vi "Read Mixed Modules at Indexes.vi"(5 "Indexes":i32[](array[numeric]), 7 "R/W Case":T1, 8 "error in (no error)":errorcluster, 10 "Async in in":T13, 11 "RSI Modules in in":T2[](array[typedef]) {"Module Config Data"."Config Block Data Refs"."Data Reference" format="%.0x"; "CDOutput Data"."BD Refs"."Data Reference" format="%.0x"; "CDInput Data"."BD Refs"."Data Reference" format="%.0x"; "VS ref" format="%.0x"}) -> (0 "error out":errorcluster, 2 "Async in out":T13, 3 "RSI Modules in out":T2[](array[typedef]) {"Module Config Data"."Config Block Data Refs"."Data Reference" format="%.0x"; "CDOutput Data"."BD Refs"."Data Reference" format="%.0x"; "CDInput Data"."BD Refs"."Data Reference" format="%.0x"; "VS ref" format="%.0x"})   [LabVIEW 2016, in "Scan Engine Custom Device.lvlib"]
uses:
  Scan Engine Custom Device.lvlib
  Type Defs/Async Command.ctl
  Type Defs/Async State.ctl
  Type Defs/Async Status.ctl
  Type Defs/Async Data.ctl
  <vilib>/NI Veristand/Custom Device API/Custom Device Item Ref.ctl
  <vilib>/NI Veristand/Custom Device API/Custom Device API.lvlib
  <vilib>/NI Veristand/Custom Device API/Data Reference.ctl
  <vilib>/NI Veristand/Custom Device API/Block Data Reference.ctl
  Type Defs/Input Data.ctl
  Type Defs/Output Data.ctl
  Modules.lvlibp/RSI Module/Channel Type.ctl
  Modules.lvlibp/RSI Module/RSI Module.lvclass
  Modules.lvlibp/RSI Module/Module Models.ctl
  Type Defs/Module Config Data.ctl
  Type Defs/Mixed IO.ctl
  Type Defs/Open Module IOVs.ctl
  Type Defs/RSI Module Data.ctl
  Type Defs/RW Case.ctl
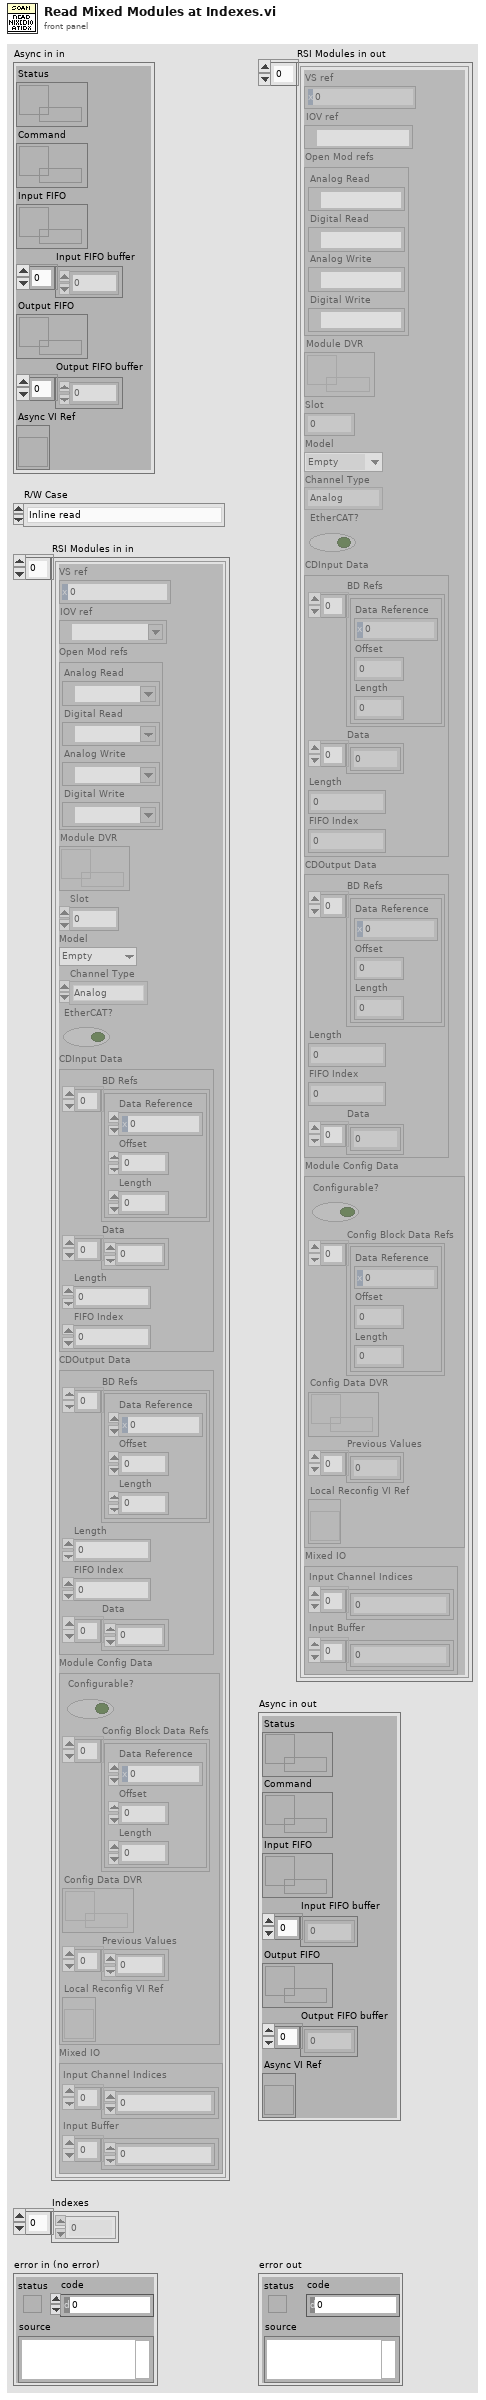
[diagram p1: front panel]
types:
  T1 = typedef "Scan Engine Custom Device.lvlib/RW Case.ctl" = enum16{"Inline read", "Inline write", "Async - Inline loop read", "Async - Inline loop write", "Async loop (read/write)"}
  T2 = typedef "Scan Engine Custom Device.lvlib/RSI Module Data.ctl" = cluster{"VS ref":T3, "IOV ref":refnum<k21>, "Open Mod refs":T4, "Module DVR":refnum<data-value>, "Slot":u32, "Model":T5, "Channel Type":T6, "EtherCAT?":bool, "CDInput Data":T7, "CDOutput Data":T10, "Module Config Data":T11, "Mixed IO":T12}
  T3 = typedef "Custom Device API.lvlib/Custom Device Item Ref.ctl" = u64
  T4 = typedef "Scan Engine Custom Device.lvlib/Open Module IOVs.ctl" = cluster{"Analog Read":refnum<k21>, "Digital Read":refnum<k21>, "Analog Write":refnum<k21>, "Digital Write":refnum<k21>}
  T5 = typedef "Modules.lvlibp/RSI Module.lvclass/Module Models.ctl" = enum16{"Empty", "NI 9201", "NI 9203", "NI 9205", "NI 9206", "NI 9207", "NI 9208", "NI 9211", "NI 9213", "NI 9214", "NI 9215", "NI 9217", "NI 9219", "NI 9221", "NI 9225", "NI 9227", "NI 9229", "NI 9233", "NI 9234", "NI 9235", "NI 9236", "NI 9237", "NI 9239", "NI 9263", "NI 9264", "NI 9265", "NI 9269", "NI 9375", "NI 9401", "NI 9402", "NI 9403", "NI 9411", "NI 9421", "NI 9422", "NI 9423", "NI 9425", "NI 9426", "NI 9435", "NI 9472", "NI 9474", "NI 9475", "NI 9476", "NI 9477", "NI 9478", "NI 9481", "NI 9482", "NI 9485"}
  T6 = typedef "Modules.lvlibp/RSI Module.lvclass/Channel Type.ctl" = enum16{"Analog", "Digital"}
  T7 = typedef "Scan Engine Custom Device.lvlib/Input Data.ctl" = cluster{"BD Refs":T8[], "Data":dbl[], "Length":i32, "FIFO Index":i32}
  T8 = typedef "Custom Device API.lvlib/Block Data Reference.ctl" = cluster{"Data Reference":T9, "Offset":u64, "Length":u64}
  T9 = typedef "Custom Device API.lvlib/Data Reference.ctl" = i32
  T10 = typedef "Scan Engine Custom Device.lvlib/Output Data.ctl" = cluster{"BD Refs":T8[], "Length":i32, "FIFO Index":i32, "Data":dbl[]}
  T11 = typedef "Scan Engine Custom Device.lvlib/Module Config Data.ctl" = cluster{"Configurable?":bool, "Config Block Data Refs":T8[], "Config Data DVR":refnum<data-value>, "Previous Values":dbl[], "Local Reconfig VI Ref":refnum<vi>}
  T12 = typedef "Scan Engine Custom Device.lvlib/Mixed IO.ctl" = cluster{"Input Channel Indices":i32[], "Input Buffer":dbl[]}
  T13 = typedef "Scan Engine Custom Device.lvlib/Async Data.ctl" = cluster{"Status":refnum<queue>, "Command":refnum<queue>, "Input FIFO":refnum<k33>, "Input FIFO buffer":dbl[], "Output FIFO":refnum<k33>, "Output FIFO buffer":dbl[], "Async VI Ref":refnum<vi>}
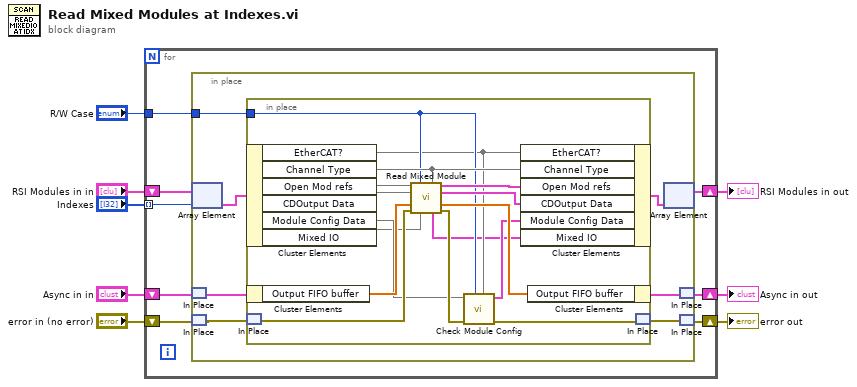
[diagram p0: block diagram]
diagram:
  n1 = for {
    shift-right: [w10] -> w4
    shift-left: "error in (no error)" -> [w11]
    shift-right: [w15] -> w2
    shift-left: "RSI Modules in in" -> [w16]
    tunnel: "R/W Case" -> [w14]
    shift-right: [w12] -> w5
    shift-left: "Async in in" -> [w13]
    tunnel: "Indexes" -> [w9] mode=indexing
    n2 = in-place {
      in-place-border: w14 -> [w21]
      n3 = in-place-array #1(w16, w9) -> (w23:T2)
      n4 = in-place-match #2(w13) -> (w20:T13)
      n5 = in-place-match #3(w11) -> (w18:errorcluster)
      n6 = in-place {
        in-place-border: w21 -> [w28]
        n7 = in-place-cluster #4(w23) -> ("EtherCAT?"=w27, "Channel Type"=w36, "Open Mod refs"=w33, "CDOutput Data"=w39, "Module Config Data"=w29, "Mixed IO"=w25)
        n8 = in-place-cluster #5(w20) -> ("Output FIFO buffer"=w35:dbl[])
        n9 = in-place-match #6(w18) -> (w31:errorcluster)
        n10 = call "Read Mixed Module.vi"("IOV ref in"=w33, "R/W Case"=w28, "Channel Type"=w36, "Output Data in"=w39, "Output FIFO buffer in"=w35, "error in (no error)"=w31, "Mixed IO in"=w25) -> ("IOV ref out"=w38:T4, "Output Data out"=w37:T10, "Output FIFO buffer out"=w34:dbl[], "Mixed IO out"=w24:T12, "error out"=w32:errorcluster)  [unwired: 4 in]
        n11 = call "Check Module Config.vi"("EtherCAT?"=w27, "R/W Case"=w28, "error in (no error)"=w32, "Module Config Data in"=w29) -> ("error out"=w30:errorcluster, "Module Config Data out"=w26:T11)  [unwired: 6 in]
        n12 = in-place-cluster #4("EtherCAT?"=w27, "Channel Type"=w36, "Open Mod refs"=w38, "CDOutput Data"=w37, "Module Config Data"=w26, "Mixed IO"=w24) -> (w22:cluster{})
        n13 = in-place-cluster #5("Output FIFO buffer"=w34) -> (w19:T13)
        n14 = in-place-match #6(w30) -> (w17:errorcluster)
      }
      n15 = in-place-array #1(w22) -> (w15:T2[])  [unwired: 1 out]
      n16 = in-place-match #2(w19) -> (w12:T13)
      n17 = in-place-match #3(w17) -> (w10:errorcluster)
    }
  }
  "Async in out" <- w5
  "error out" <- w4
  "RSI Modules in out" <- w2
